vi "Hardware-NOxDataCalPoints.vi"(9 "NOx Sensor Data 2":T1 {"Sensor Supply Status" items=["NOT IN RANGE", "SUPPLY IN RANGE", "ERROR", "NOT AVAILABLE"]; "Sensor Temperature Status" items=["NOT AT TEMPERATURE"=0, "AT TEMPERATURE"=4, "ERROR"=8, "NOT AVAILABLE"=12]; "NOx Signal Status" items=["NOT VALID"=0, "VALID"=16, "ERROR"=32, "NOT AVAILABLE"=48]; "O2 Signal Status" items=["NOT VALID"=0, "VALID"=64, "ERROR"=128, "NOT AVAILABLE"=192]; "Heater Mode Status" items=["AUTO MODE"=0, "HEATUP SLOPE 3 OR 4"=32, "HEATUP SLOPE 1 OR 2"=64, "HEATER OFF / PREHEAT"=96]; "Heater Circuit Status" items=["OPEN WIRE"=3, "SHORT CIRCUIT"=5, "NO ERROR"=31]; "NOx Circuit Status" items=["OPEN WIRE"=3, "SHORT CIRCUIT"=5, "NO ERROR"=31]; "O2 Circuit Status" items=["OPEN WIRE"=3, "SHORT CIRCUIT"=5, "NO ERROR"=31]; "O2 [%}" format="%#_3p"; "NOx [ppm]" format="%#_3p"}, 10 "NOx Sensor Data":T1 {"Sensor Supply Status" items=["NOT IN RANGE", "SUPPLY IN RANGE", "ERROR", "NOT AVAILABLE"]; "Sensor Temperature Status" items=["NOT AT TEMPERATURE"=0, "AT TEMPERATURE"=4, "ERROR"=8, "NOT AVAILABLE"=12]; "NOx Signal Status" items=["NOT VALID"=0, "VALID"=16, "ERROR"=32, "NOT AVAILABLE"=48]; "O2 Signal Status" items=["NOT VALID"=0, "VALID"=64, "ERROR"=128, "NOT AVAILABLE"=192]; "Heater Mode Status" items=["AUTO MODE"=0, "HEATUP SLOPE 3 OR 4"=32, "HEATUP SLOPE 1 OR 2"=64, "HEATER OFF / PREHEAT"=96]; "Heater Circuit Status" items=["OPEN WIRE"=3, "SHORT CIRCUIT"=5, "NO ERROR"=31]; "NOx Circuit Status" items=["OPEN WIRE"=3, "SHORT CIRCUIT"=5, "NO ERROR"=31]; "O2 Circuit Status" items=["OPEN WIRE"=3, "SHORT CIRCUIT"=5, "NO ERROR"=31]; "O2 [%}" format="%#_3p"; "NOx [ppm]" format="%#_3p"}) -> ()   [LabVIEW 2015, in "DSI-RT.lvlib"]
uses:
  DSI-RT.lvlib
  <vilib>/Powertrain Controls/Device Drivers/DCM/Tools/RT/NOx Data.ctl
  <vilib>/Powertrain Controls/Device Drivers/DCM/Tools/RT/DCM - RT - Tools.lvlib
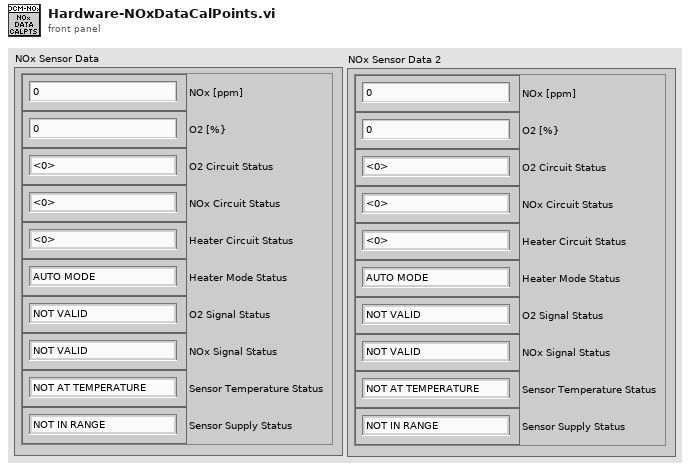
[diagram p1: front panel]
types:
  T1 = typedef "DCM - RT - Tools.lvlib/NOx Data.ctl" = cluster{"NOx [ppm]":sgl, "O2 [%}":sgl, "O2 Circuit Status":u8, "NOx Circuit Status":u8, "Heater Circuit Status":u8, "Heater Mode Status":u8, "O2 Signal Status":u8, "NOx Signal Status":u8, "Sensor Temperature Status":u8, "Sensor Supply Status":u8}
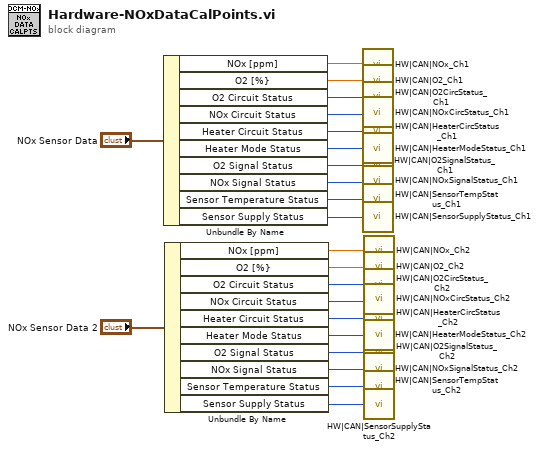
[diagram p0: block diagram]
diagram:
  n1 = Unbundle By Name("NOx Sensor Data") -> ("NOx [ppm]"=w21:sgl, "O2 [%}"=w20:sgl, "O2 Circuit Status"=w19:u8, "NOx Circuit Status"=w18:u8, "Heater Circuit Status"=w17:u8, "Heater Mode Status"=w16:u8, "O2 Signal Status"=w15:u8, "NOx Signal Status"=w14:u8, "Sensor Temperature Status"=w13:u8, "Sensor Supply Status"=w12:u8)
  n2 = Unbundle By Name("NOx Sensor Data 2") -> ("NOx [ppm]"=w2:sgl, "O2 [%}"=w3:sgl, "O2 Circuit Status"=w4:u8, "NOx Circuit Status"=w5:u8, "Heater Circuit Status"=w6:u8, "Heater Mode Status"=w7:u8, "O2 Signal Status"=w8:u8, "NOx Signal Status"=w9:u8, "Sensor Temperature Status"=w10:u8, "Sensor Supply Status"=w11:u8)
  n3 = call "HW|CAN|NOx_Ch1"("Value"=w21) -> ()
  n4 = call "HW|CAN|O2_Ch1"("Value"=w20) -> ()
  n5 = call "HW|CAN|O2CircStatus_Ch1"("Value"=w19) -> ()
  n6 = call "HW|CAN|NOxCircStatus_Ch1"("Value"=w18) -> ()
  n7 = call "HW|CAN|HeaterCircStatus_Ch1"("Value"=w17) -> ()
  n8 = call "HW|CAN|HeaterModeStatus_Ch1"("Value"=w16) -> ()
  n9 = call "HW|CAN|O2SignalStatus_Ch1"("Value"=w15) -> ()
  n10 = call "HW|CAN|NOxSignalStatus_Ch1"("Value"=w14) -> ()
  n11 = call "HW|CAN|SensorTempStatus_Ch1"("Value"=w13) -> ()
  n12 = call "HW|CAN|SensorSupplyStatus_Ch1"("Value"=w12) -> ()
  n13 = call "HW|CAN|NOx_Ch2"("Value"=w2) -> ()
  n14 = call "HW|CAN|O2_Ch2"("Value"=w3) -> ()
  n15 = call "HW|CAN|O2CircStatus_Ch2"("Value"=w4) -> ()
  n16 = call "HW|CAN|NOxCircStatus_Ch2"("Value"=w5) -> ()
  n17 = call "HW|CAN|HeaterCircStatus_Ch2"("Value"=w6) -> ()
  n18 = call "HW|CAN|HeaterModeStatus_Ch2"("Value"=w7) -> ()
  n19 = call "HW|CAN|O2SignalStatus_Ch2"("Value"=w8) -> ()
  n20 = call "HW|CAN|NOxSignalStatus_Ch2"("Value"=w9) -> ()
  n21 = call "HW|CAN|SensorTempStatus_Ch2"("Value"=w10) -> ()
  n22 = call "HW|CAN|SensorSupplyStatus_Ch2"("Value"=w11) -> ()
